vi "QPSK.vi"(8 "ebn0":dbl=10.0) -> (0 "Pr(error) ideal":dbl=3.8721082155220345e-06, 1 "Pr(error) measured":dbl=4.417309341754243e-06, 2 "Histogram (cos)":dynamicdata(graph)=[{"t0"=timestamp(-1.485 s since 1904-01-01), "dt"=0.03, "Y"=[0.0, 0.0, 0.0, 0.0, 0.0, 0.0, 0.0, 0.0, 0.0, 0.0, 0.0, 0.0, 0.0, 0.0, 0.0, 0.0, 0.0, 0.0, 0.0, 0.0, 0.0, 0.0, 0.0, 0.0, 0.0, 0.0, 0.0, 0.0, 0.0, 0.0, 0.0, 0.0, 0.0, 0.0, 3.4241333604068144e-05, 3.4241333604068144e-05, 0.0, 6.848266720813629e-05, 0.00013696533441627257, 3.4241333604068144e-05, 3.4241333604068144e-05, 0.00013696533441627257, 0.00017120666802034073, 0.00017120666802034073, 0.0003081720024366133, 0.00034241333604068146, 0.0005136200040610221, 0.0005478613376650903, 0.0010272400081220443, 0.0015066186785789983, 0.0019517560154318843, 0.003115961357970201, 0.004554097369341063, 0.0058210267126915845, 0.009279401406702466, 0.013662292108023189, 0.020510558828836817, 0.02948178823310267, 0.04156897899533873, 0.05961416180468264, 0.08519243800692154, 0.12046101161911173, 0.1656253306428776, 0.22904028047761182, 0.3093362077791516, 0.4193536126490226, 0.5559422923956504, 0.7109185682876629, 0.9207152192797883, 1.1575282824855235, 1.4447445887564472, 1.7548683472084925, 2.1085470820049124, 2.4922212250384956, 2.891269726860306, 3.3243883556181637, 3.747371549629218, 4.118718812565337, 4.4982155128992245, 4.799607731282231, 5.035633243815074, 5.185610285000892, 5.283814429777359, 5.297750652554215, 5.198690474437646, 4.992797335476384, 4.7311593054077, 4.398573232111386, 4.044997221315778, 3.6019143644791365, 3.2011880373107267, 2.7670079272111425, 2.3564200959647614, 1.9809296316625504, 1.6277645168701913, 1.3070944276680934, 1.038676613545803, 0.8117935370852475, 0.6223019969203345, 0.4671887556939058], "attributes"=variant("NI_ChannelName"=variant(string " (Histogram)"), "NI_ExpIsRelativeTime"=variant(bool TRUE), "NI_ExpStartTimeStamp"=variant(timestamp timestamp(0 s since 1904-01-01)), "NI_ExpTimeStamp"=variant(timestamp timestamp(0 s since 1904-01-01)), "NI_ExpXDimension"=variant(string "BIN"), "NI_OriginalChannelName"=variant(string ""))}, {"t0"=timestamp(-1.485 s since 1904-01-01), "dt"=0.03, "Y"=[0.4605704235267759, 0.6244627848888776, 0.8202154924187792, 1.0258003712929373, 1.3087750587617837, 1.6241239689495233, 1.9662629766676063, 2.364003427214011, 2.7824359735511166, 3.1896317526376428, 3.6130317723019854, 4.009573177562506, 4.38264755365642, 4.73061049562023, 5.009063069439454, 5.192996616294203, 5.330955341044451, 5.295840443386392, 5.213346127717507, 5.04112896622769, 4.806390157688158, 4.492925461521096, 4.142119069307901, 3.7189246002639953, 3.3040206729110664, 2.883395586622629, 2.490245766599326, 2.1102854447207577, 1.756087467270346, 1.4409783661397833, 1.158723105842468, 0.9185029474246049, 0.7158985525467892, 0.5552950011116863, 0.4162742648225122, 0.3077435372315552, 0.22925745866120084, 0.16896260999955806, 0.11993878702523374, 0.08663958651437192, 0.056423645310071394, 0.04100734877726501, 0.028605794677540753, 0.019938410182429603, 0.013771891569307044, 0.009421070103381685, 0.007365563899007499, 0.003871203351571383, 0.003699911167873534, 0.002774933375905151, 0.0012675621593640812, 0.0012333037226245115, 0.00047961811435397666, 0.0005823934245726859, 0.00044535967761440696, 0.00041110124087483715, 0.00017129218369784882, 0.00010277531021870929, 6.851687347913953e-05, 0.00017129218369784882, 3.4258436739569764e-05, 3.4258436739569764e-05, 0.0, 0.0, 3.4258436739569764e-05, 0.0, 0.0, 0.0, 0.0, 0.0, 0.0, 0.0, 0.0, 0.0, 0.0, 0.0, 0.0, 0.0, 0.0, 0.0, 0.0, 0.0, 0.0, 0.0, 0.0, 0.0, 0.0, 0.0, 0.0, 0.0, 0.0, 0.0, 0.0, 0.0, 0.0, 0.0, 0.0, 0.0, 0.0, 0.0], "attributes"=variant("NI_ChannelName"=variant(string " (Histogram)"), "NI_ExpIsRelativeTime"=variant(bool TRUE), "NI_ExpStartTimeStamp"=variant(timestamp timestamp(0 s since 1904-01-01)), "NI_ExpTimeStamp"=variant(timestamp timestamp(0 s since 1904-01-01)), "NI_ExpXDimension"=variant(string "BIN"), "NI_OriginalChannelName"=variant(string ""))}] caption="Histogram", 3 "Histogram (sin)":dynamicdata(graph)=[{"t0"=timestamp(-1.485 s since 1904-01-01), "dt"=0.03, "Y"=[0.0, 0.0, 0.0, 0.0, 0.0, 0.0, 0.0, 0.0, 0.0, 0.0, 0.0, 0.0, 0.0, 0.0, 0.0, 0.0, 0.0, 0.0, 0.0, 0.0, 0.0, 0.0, 0.0, 0.0, 0.0, 0.0, 0.0, 0.0, 0.0, 0.0, 0.0, 0.0, 0.0, 3.4260455520164504e-05, 0.0, 0.0, 0.0, 3.4260455520164504e-05, 3.4260455520164504e-05, 6.852091104032901e-05, 3.4260455520164504e-05, 0.00017130227760082253, 0.00023982318864115154, 0.00017130227760082253, 0.00034260455520164506, 0.0004796463772823031, 0.0004796463772823031, 0.0009592927545646062, 0.0009592927545646062, 0.001952845964649377, 0.0025695341640123376, 0.002398231886411515, 0.004762203317302866, 0.005961319260508624, 0.008839197524202442, 0.012984712642142349, 0.01908307372473163, 0.028847303547978514, 0.042140360289802344, 0.062319768591179235, 0.08496592969000798, 0.12422841171611648, 0.171610621700504, 0.23197754432703385, 0.3131063029987834, 0.4176692132463255, 0.5488182369775152, 0.7202575564004183, 0.9136235673562267, 1.1599219820906896, 1.4304767993334286, 1.7611244555585361, 2.1043114385040242, 2.4651425560423967, 2.902100405746575, 3.3358377726318578, 3.731888638444959, 4.110192588298616, 4.49634218246639, 4.828154694179183, 5.024021718387963, 5.2148867160908, 5.285531775373379, 5.273060969564039, 5.178090986862143, 4.991508546099327, 4.732807846466565, 4.3975007682907155, 4.028310099605422, 3.6242765476561223, 3.1807406904920725, 2.775336720321966, 2.3553377961002693, 1.9992346214236796, 1.6298041295497456, 1.3092975681586068, 1.0476162088955903, 0.8131376513155844, 0.6244653227660385, 0.46741539466160437], "attributes"=variant("NI_ChannelName"=variant(string " (Histogram)"), "NI_ExpIsRelativeTime"=variant(bool TRUE), "NI_ExpStartTimeStamp"=variant(timestamp timestamp(0 s since 1904-01-01)), "NI_ExpTimeStamp"=variant(timestamp timestamp(0 s since 1904-01-01)), "NI_ExpXDimension"=variant(string "BIN"), "NI_OriginalChannelName"=variant(string ""))}, {"t0"=timestamp(-1.485 s since 1904-01-01), "dt"=0.03, "Y"=[0.4668814531411237, 0.6228168445841649, 0.816391813272078, 1.0426060150030876, 1.3106724127243006, 1.6264475739597144, 1.9750674618355577, 2.3604364547011625, 2.7679302582129797, 3.1913498155181226, 3.6046316886881598, 4.017399827864863, 4.406262211885133, 4.732243555121431, 4.980274327102653, 5.17525350203901, 5.289062706028737, 5.2729314586380776, 5.242210165836758, 5.064081465881727, 4.809372151987175, 4.4875691785633185, 4.128092378961703, 3.738579265216544, 3.297110520278965, 2.9053369769631403, 2.4834243727051075, 2.117988258780827, 1.7592991846356547, 1.4269132909491373, 1.163812988496811, 0.9222552648315859, 0.707548704551238, 0.5538052448130848, 0.418624706700701, 0.3150559336447475, 0.22823488877145312, 0.16689504996748064, 0.12113847562794562, 0.08521134502751732, 0.0605178644146395, 0.045003097815979796, 0.028769103626653754, 0.021028844793768337, 0.014076311417327014, 0.008253992826218517, 0.006438799383108222, 0.0047606016715534185, 0.0029796571613319956, 0.0019521891746657903, 0.0014384551813326875, 0.0010617169195550789, 0.0008562233222218378, 0.00047948506044422925, 0.0005137339933331027, 0.00013699573155549408, 0.00017124466444436758, 0.00010274679866662055, 6.849786577774704e-05, 3.424893288887352e-05, 3.424893288887352e-05, 0.0, 0.00010274679866662055, 0.0, 0.0, 0.0, 0.0, 0.0, 0.0, 0.0, 0.0, 0.0, 0.0, 0.0, 0.0, 0.0, 0.0, 0.0, 0.0, 0.0, 0.0, 0.0, 0.0, 0.0, 0.0, 0.0, 0.0, 0.0, 0.0, 0.0, 0.0, 0.0, 0.0, 0.0, 0.0, 0.0, 0.0, 0.0, 0.0, 0.0], "attributes"=variant("NI_ChannelName"=variant(string " (Histogram)"), "NI_ExpIsRelativeTime"=variant(bool TRUE), "NI_ExpStartTimeStamp"=variant(timestamp timestamp(0 s since 1904-01-01)), "NI_ExpTimeStamp"=variant(timestamp timestamp(0 s since 1904-01-01)), "NI_ExpXDimension"=variant(string "BIN"), "NI_OriginalChannelName"=variant(string ""))}] caption="Histogram", 6 "Sigma_out (measured)":dbl=0.2235617892354569 format="%.6f", 7 "Sigma_out (Ideal)":dbl=0.22360679774997896)   [LabVIEW 2019]
uses:
  <vilib>/imath/engines/lvmath2/RunTimeEngine/NodeEndStatement/NIMS_NodeEndStatement_Output.vi
  <instcachedir>/0/NIMS_NodeEndStatement_Output_53EC0D466D134D7ABD903AC30B43404B.lvgen/NIMS_NodeEndStatement_Output_53EC0D466D134D7ABD903AC30B43404B_009.vi
  <vilib>/imath/engines/lvmath2/RunTimeEngine/ErrorHandling/NIMS_Finalize Error.vi
  <vilib>/measure/NI_MABase.lvlib
  <vilib>/gmath/NI_Gmath.lvlib
  <vilib>/Analysis/NI_AALBase.lvlib
panel:
  out "Graphs (sin)":waveform(dbl)[](graph)=[{"t0"=timestamp(0 s since 1904-01-01), "dt"=0.01, "Y"=array[1000 elements]}, {"t0"=timestamp(0 s since 1904-01-01), "dt"=0.01, "Y"=array[1000 elements]}, {"t0"=timestamp(0 s since 1904-01-01), "dt"=0.01, "Y"=array[1000 elements], "attributes"=variant("NI_ChannelName"=variant(string "Integral (Sum[Xdt])"))}]
  out "I_out (sin)":dbl=-0.8304582234845936
  out "s(t) amplitude":dbl=0.2
  in  "s":dbl=1000.0
  in  "sigma_in 2":dbl=1.0
  out "T":dbl=10.0
  out "E_b":dbl=0.20000000000000004
  out "E_b / N_0 (dB)":dbl=10.0
  out "E_b / N_0":dbl=10.000000000000002
  out "N_0":dbl=0.02
  in  "sampling info":cluster{"Fs":dbl, "#s":dbl}={"Fs"=100.0, "#s"=1000.0} {"Fs" format="%.2p"}
  out "Graphs (cos)":waveform(dbl)[](graph)=[{"t0"=timestamp(0 s since 1904-01-01), "dt"=0.01, "Y"=array[1000 elements]}, {"t0"=timestamp(0 s since 1904-01-01), "dt"=0.01, "Y"=array[1000 elements]}, {"t0"=timestamp(0 s since 1904-01-01), "dt"=0.01, "Y"=array[1000 elements], "attributes"=variant("NI_ChannelName"=variant(string "Integral (Sum[Xdt])"))}]
  out "I_out (cos)":dbl=1.086309838008856
  in  "oscillator frequency":dbl=1.0 format="%0.2p"
  in  "oscillator amplitude":dbl=1.0 format="%0.2p"
  in  "s(t) frequency":dbl=1.0 format="%0.2p"
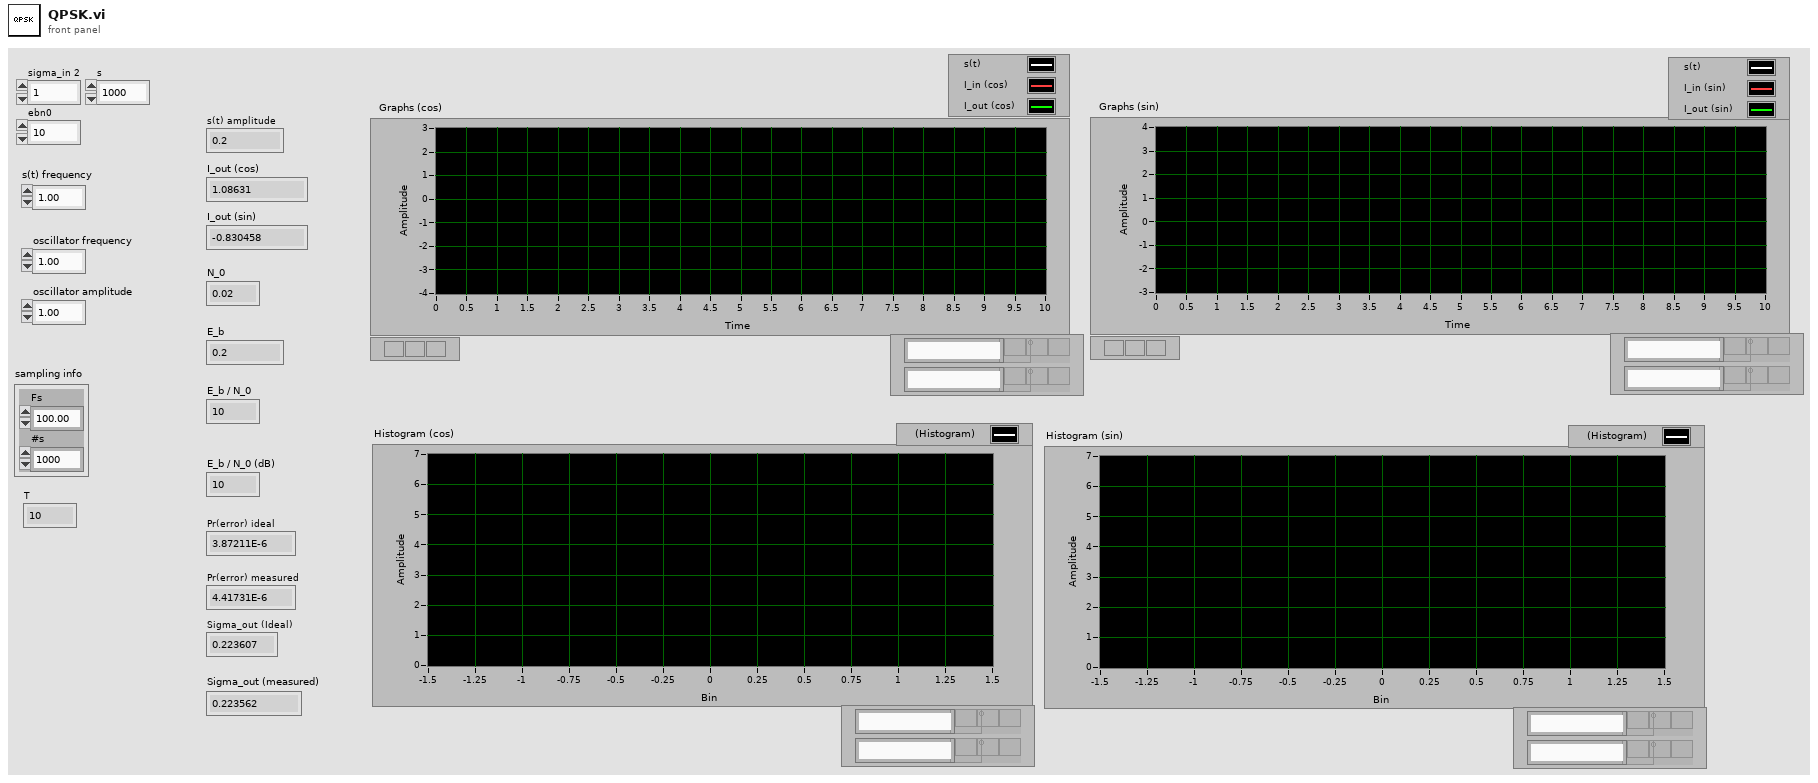
[diagram p1: front panel]
types:
  T1 = enum16{"Sine Wave", "Triangle Wave", "Square Wave", "Sawtooth Wave"}
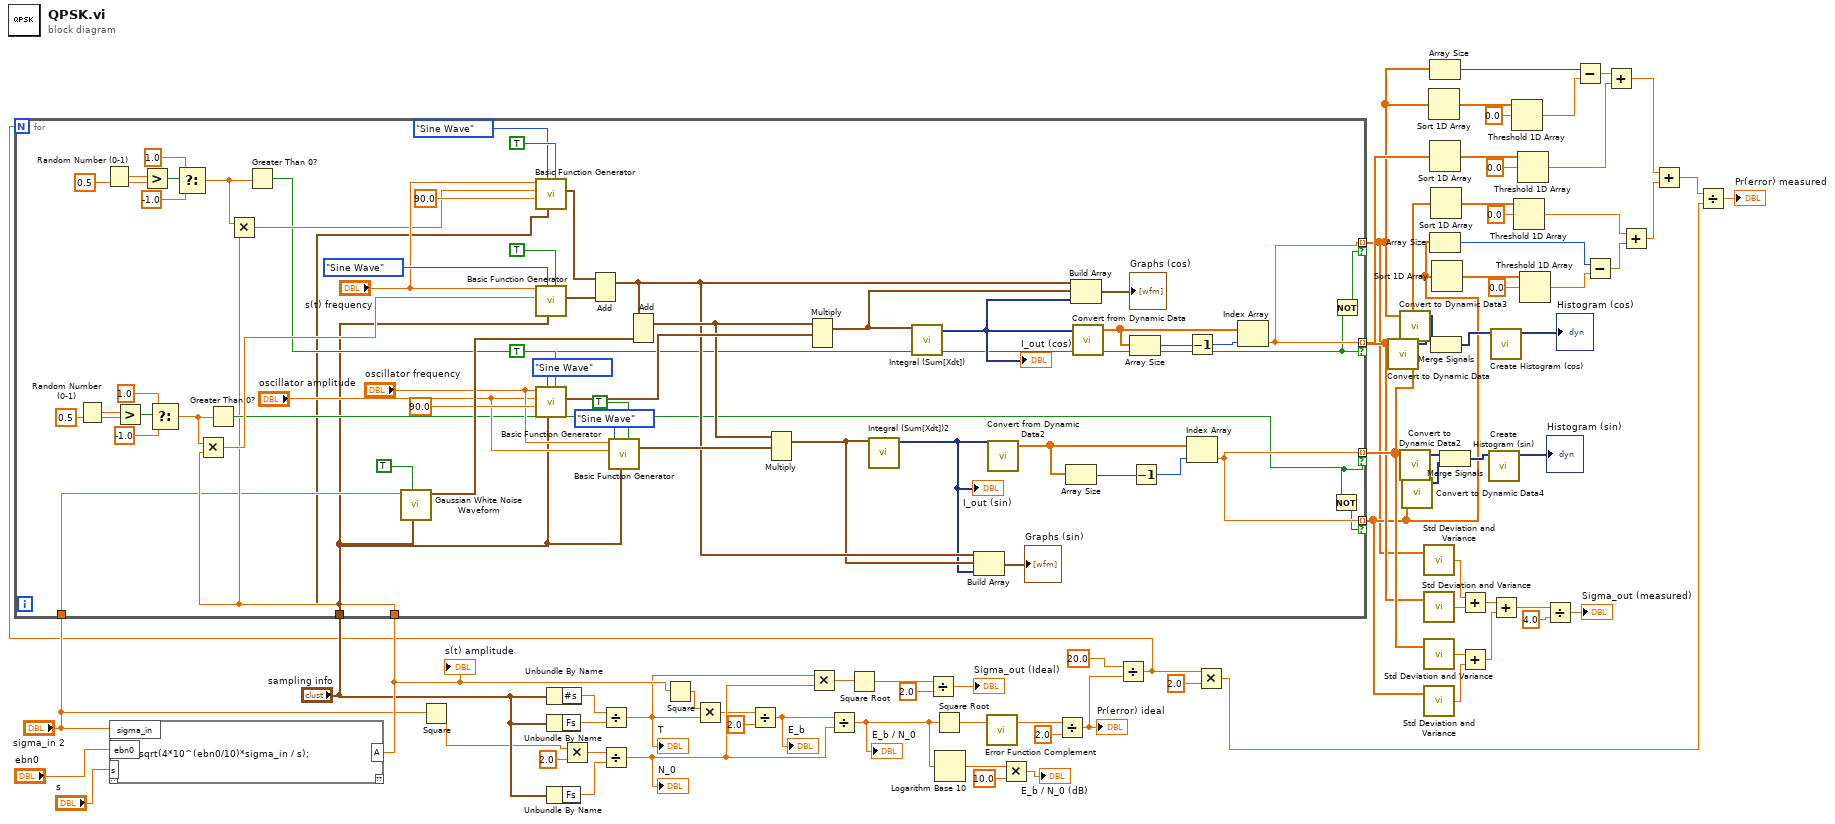
[diagram p0: block diagram]
diagram:
  n1 = mathscript code="A = sqrt(4*10^(ebn0/10)*sigma_in / s);"("s"="s", "ebn0"="ebn0", "sigma_in"="sigma_in 2") -> ("A"=w33:cdb)  [unwired: 1 in, 1 out]
  "s(t) amplitude" <- w33
  n2 = Square(x="sigma_in 2") -> (x^2=w7:dbl)
  n3 = Unbundle By Name("sampling info") -> ("#s"=w24:dbl)
  n4 = Unbundle By Name("sampling info") -> ("Fs"=w14:dbl)
  n5 = Unbundle By Name("sampling info") -> ("Fs"=w19:dbl)
  n6 = Multiply(x=w7, y=2.0) -> (x*y=w20:dbl)
  n7 = Divide(x=w24, y=w14) -> (x/y=w6:dbl)
  "T" <- w6
  n8 = Divide(x=w20, y=w19) -> (x/y=w29:dbl)
  "N_0" <- w29
  n9 = Square(x=w33) -> (x^2=w17:cdb)
  n10 = Multiply(x=w17, y=w6) -> (x*y=w16:cdb)
  n11 = Divide(x=w16, y=2.0) -> (x/y=w15:cdb)
  "E_b" <- w15
  n12 = Multiply(x=w6, y=w29) -> (x*y=w26:dbl)
  n13 = Divide(x=w15, y=w29) -> (x/y=w25:cdb)
  "E_b / N_0" <- w25
  n14 = Square Root(x=w26) -> (sqrt(x)=w27:dbl)
  n15 = Divide(x=w27, y=2.0) -> (x/y=→"Sigma_out (Ideal)":dbl)
  n16 = Square Root(x=w25) -> (sqrt(x)=w22:cdb)
  n17 = Logarithm Base 10(1:w25) -> (0:w18:cdb)
  n18 = call <vilib>:"Error Function Complement.vi"("x"=w22) -> ("1 - erf(x)"=w23:dbl)  [unwired: 2 in]
  n19 = Multiply(x=w18, y=10.0) -> (x*y=→"E_b / N_0 (dB)":cdb)
  n20 = Divide(x=w23, y=2.0) -> (x/y=w4:dbl)
  "Pr(error) ideal" <- w4
  n21 = Divide(x=20.0, y=w4) -> (x/y=w2:dbl)
  n22 = for {
    N: w2 -> [_]
    tunnel: [w80] -> w42 mode=indexing if=w79
    tunnel: [w83] -> w49 mode=indexing if=w82
    tunnel: [w83] -> w40 mode=indexing if=w81
    tunnel: [w80] -> w37 mode=indexing if=w78
    tunnel: w33 -> [w77]
    tunnel: "sigma_in 2" -> [w76]
    tunnel: "sampling info" -> [w75]
    n23 = Random Number (0-1)() -> (number: 0 to 1=w100:dbl)
    n24 = Random Number (0-1)() -> (number: 0 to 1=w104:dbl)
    n25 = Greater?(x=w100, y=0.5) -> (0:w99:bool)
    n26 = Greater?(x=w104, y=0.5) -> (0:w103:bool)
    n27 = Select(t=1.0, s=w99, f=-1.0) -> (s? t:f=w86:dbl)
    n28 = Select(t=1.0, s=w103, f=-1.0) -> (s? t:f=w87:dbl)
    n29 = Multiply(x=w86, y=w77) -> (x*y=w85:cdb)
    n30 = Greater Than 0?(x=w86) -> (x > 0?=w82:bool)
    n31 = Multiply(x=w87, y=w77) -> (x*y=w84:cdb)
    n32 = Greater Than 0?(x=w87) -> (x > 0?=w79:bool)
    n33 = call <vilib>:"Gaussian White Noise Waveform.vi"("sampling info"=w75, "reset signal"=TRUE, "standard deviation"=w76) -> ("signal out"=w124:waveform(dbl))  [unwired: 7 in, 1 out]
    n34 = call <vilib>:"Basic Function Generator.vi"("reset signal"=TRUE, "sampling info"=w75, "signal type"=T1."Sine Wave", "phase"=90.0, "amplitude"=w84, "frequency"="s(t) frequency") -> ("signal out"=w122:waveform(dbl))  [unwired: 3 in, 2 out]
    n35 = call <vilib>:"Basic Function Generator.vi"("reset signal"=TRUE, "sampling info"=w75, "signal type"=T1."Sine Wave", "amplitude"=w85, "frequency"="s(t) frequency") -> ("signal out"=w123:waveform(dbl))  [unwired: 4 in, 2 out]
    n36 = call <vilib>:"Basic Function Generator.vi"("reset signal"=TRUE, "sampling info"=w75, "signal type"=T1."Sine Wave", "phase"=90.0, "amplitude"="oscillator amplitude", "frequency"="oscillator frequency") -> ("signal out"=w125:waveform(dbl))  [unwired: 3 in, 2 out]
    n37 = Add(1:w123, 2:w122) -> (0:w94:waveform(dbl))  [unwired: 1 in, 1 out]
    n38 = call <vilib>:"Basic Function Generator.vi"("reset signal"=TRUE, "sampling info"=w75, "signal type"=T1."Sine Wave" ("oscillator (sin)"), "amplitude"="oscillator amplitude", "frequency"="oscillator frequency") -> ("signal out"=w111:waveform(dbl))  [unwired: 4 in, 2 out]
    n39 = Add(1:w124, 2:w94) -> (0:w112:waveform(dbl))  [unwired: 1 in, 1 out]
    n40 = Multiply(1:w111, 2:w112) -> (0:w93:waveform(dbl))  [unwired: 1 in, 1 out]
    n41 = Multiply(1:w125, 2:w112) -> (0:w126:waveform(dbl))  [unwired: 1 in, 1 out]
    n42 = call "Integral (Sum[Xdt])2"("Signals"=w93) -> ("Result"=w92:dynamicdata)  [unwired: 5 in, 1 out]
    "I_out (sin)" <- w92
    n43 = call "Integral (Sum[Xdt])"("Signals"=w126) -> ("Result"=w96:dynamicdata)  [unwired: 5 in, 1 out]
    "I_out (cos)" <- w96
    n44 = Build Array(w94, w93, w92) -> (→"Graphs (sin)":waveform(dbl)[])
    n45 = call "Convert from Dynamic Data2"("Dynamic Data Type"=w92) -> ("Array"=w107:dbl[])  [unwired: 3 in]
    n46 = Array Size(array=w107) -> (size(s)=w106:i32)
    n47 = Build Array(w94, w126, w96) -> (→"Graphs (cos)":waveform(dbl)[])
    n48 = call "Convert from Dynamic Data"("Dynamic Data Type"=w96) -> ("Array"=w128:dbl[])  [unwired: 3 in]
    n49 = Array Size(array=w128) -> (size(s)=w129:i32)
    n50 = Decrement(x=w106) -> (x-1=w105:i32)
    n51 = Decrement(x=w129) -> (x-1=w130:i32)
    n52 = Index Array(array=w107, index=w105) -> (element=w83:dbl)
    n53 = Index Array(array=w128, index=w130) -> (element=w80:dbl)
    n54 = Not(x=w82) -> (.not. x?=w81:bool)
    n55 = Not(x=w79) -> (.not. x?=w78:bool)
  }
  n56 = Multiply(x=w2, y=2.0) -> (x*y=w1:dbl)
  n57 = call "Convert to Dynamic Data"("Array"=w42) -> ("Dynamic Data Type"=w73:dynamicdata)  [unwired: 3 in]
  n58 = call "Convert to Dynamic Data3"("Array"=w37) -> ("Dynamic Data Type"=w69:dynamicdata)  [unwired: 3 in]
  n59 = call "Convert to Dynamic Data2"("Array"=w49) -> ("Dynamic Data Type"=w72:dynamicdata)  [unwired: 3 in]
  n60 = call "Convert to Dynamic Data4"("Array"=w40) -> ("Dynamic Data Type"=w67:dynamicdata)  [unwired: 3 in]
  n61 = call <vilib>:"Std Deviation and Variance.vi"("X"=w37) -> ("standard deviation"=w66:dbl)  [unwired: 1 in, 2 out]
  n62 = call <vilib>:"Std Deviation and Variance.vi"("X"=w42) -> ("standard deviation"=w65:dbl)  [unwired: 1 in, 2 out]
  n63 = call <vilib>:"Std Deviation and Variance.vi"("X"=w49) -> ("standard deviation"=w63:dbl)  [unwired: 1 in, 2 out]
  n64 = call <vilib>:"Std Deviation and Variance.vi"("X"=w40) -> ("standard deviation"=w62:dbl)  [unwired: 1 in, 2 out]
  n65 = Sort 1D Array(array=w37) -> (sorted array=w57:dbl[])
  n66 = Array Size(array=w37) -> (size(s)=w41:i32)
  n67 = Sort 1D Array(array=w42) -> (sorted array=w55:dbl[])
  n68 = Array Size(array=w40) -> (size(s)=w38:i32)
  n69 = Sort 1D Array(array=w49) -> (sorted array=w53:dbl[])
  n70 = Merge Signals(w73, w69) -> (w70:dynamicdata)
  n71 = Sort 1D Array(array=w40) -> (sorted array=w51:dbl[])
  n72 = Merge Signals(w72, w67) -> (w68:dynamicdata)
  n73 = Add(x=w66, y=w65) -> (x+y=w61:dbl)
  n74 = Add(x=w63, y=w62) -> (x+y=w60:dbl)
  n75 = call "Create Histogram (sin)"("Signal"=w68) -> ("Histogram"=→"Histogram (sin)":dynamicdata)  [unwired: 9 in, 1 out]
  n76 = call "Create Histogram (cos)"("Signal"=w70) -> ("Histogram"=→"Histogram (cos)":dynamicdata)  [unwired: 9 in, 1 out]
  n77 = Add(x=w61, y=w60) -> (x+y=w59:dbl)
  n78 = Threshold 1D Array(2:0.0 ("threshold y"), 3:w57) -> (0:w36:dbl)  [unwired: 1 in]
  n79 = Threshold 1D Array(2:0.0 ("threshold y"), 3:w53) -> (0:w39:dbl)  [unwired: 1 in]
  n80 = Threshold 1D Array(2:0.0 ("threshold y"), 3:w55) -> (0:w34:dbl)  [unwired: 1 in]
  n81 = Threshold 1D Array(2:0.0 ("threshold y"), 3:w51) -> (0:w44:dbl)  [unwired: 1 in]
  n82 = Divide(x=w59, y=4.0) -> (x/y=→"Sigma_out (measured)":dbl)
  n83 = Subtract(x=w41, y=w36) -> (x-y=w35:dbl)
  n84 = Subtract(x=w38, y=w44) -> (x-y=w43:dbl)
  n85 = Add(x=w35, y=w34) -> (x+y=w47:dbl)
  n86 = Add(x=w39, y=w43) -> (x+y=w48:dbl)
  n87 = Add(x=w47, y=w48) -> (x+y=w46:dbl)
  n88 = Divide(x=w46, y=w1) -> (x/y=→"Pr(error) measured":dbl)
